vi "TDC_calcHbtG2_.vi"(8 "Error In":errorcluster, 11 "fct in":u64) -> (0 "Error Out":errorcluster, 3 "fct out":i32)   [LabVIEW 2011]
uses:
  tdcbase.dll
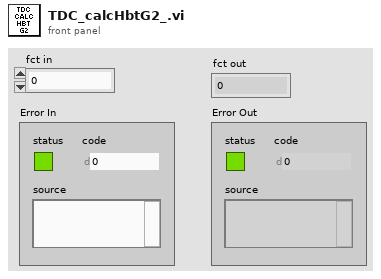
[diagram p1: front panel]
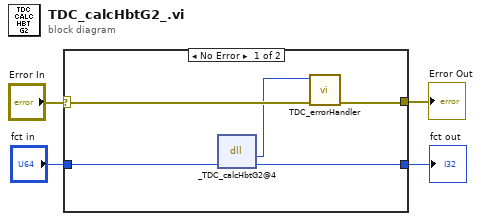
[diagram p0: block diagram]
diagram:
  n1 = case shown="No Error" "Error In" {
    selector: "Error In" -> [w7 w11]
    tunnel: [w6 w11] -> w3
    tunnel: [w9 w10] -> w2
    tunnel: "fct in" -> [w8 w10]
    frame No Error {
      n2 = dll-call lib="X:/tdcbase.dll" fn="_TDC_calcHbtG2@4"("fct"=w8) -> ("return type"=w5:i32, "fct"=w9:u64)  [unwired: 3 in, 2 out]
      n3 = call "TDC_errorHandler.vi"("Error In"=w7, "TDC Return Code"=w5) -> ("Error Out"=w6:errorcluster)  [unwired: 9 in]
    }
    frame Error {
    }
  }
  "Error Out" <- w3
  "fct out" <- w2
